vi "BorowskiMonitor.vi"() -> ()   [LabVIEW 2019]
uses:
  Utility/Monitor Communication/Brosowski/TempErrors.ctl
  Utility/Monitor Communication/Brosowski/TempErrors_in.ctl
  Utility/Monitor Communication/Brosowski/BorowskiMonitor.ctl
  Equipment/Mercury iXX/Public/Controls/Serial Settings.ctl
  Instrument_Setup.vi
  Equipment/Mercury iXX/Public/Libraries/System/Open/Open System.vi
  Global/Global Variables/Data_Display_global.vi
  Equipment/Mercury iXX/Mercury iXX.lvlib
  Equipment/Mercury iXX/Public/Libraries/Temperature.lvlib
  Equipment/Mercury iXX/Public/Libraries/Control Loop.lvlib
  Equipment/Mercury iXX/Public/Libraries/System.lvlib
panel:
  out "Borowski ITC-Cluster":T1 {"He3-Pot Heater %" format="%#_4g"; "He3-Pot Setpoint" format="%#_4g"; "Sorb Heater %" format="%#_4g"; "Sorb Setpoint" format="%#_4g"; "He3 Temp2" format="%#_4g"; "He3 Temp 1" format="%#_4g"; "1K Temp" format="%#_4g"; "Sorb Temp" format="%#_4g"}
  in  "Stop Monitoring":bool
  in  "TempErrorsIn":T2
  out "TempErrorsOut":T3
  in  "error in (no error)":errorcluster
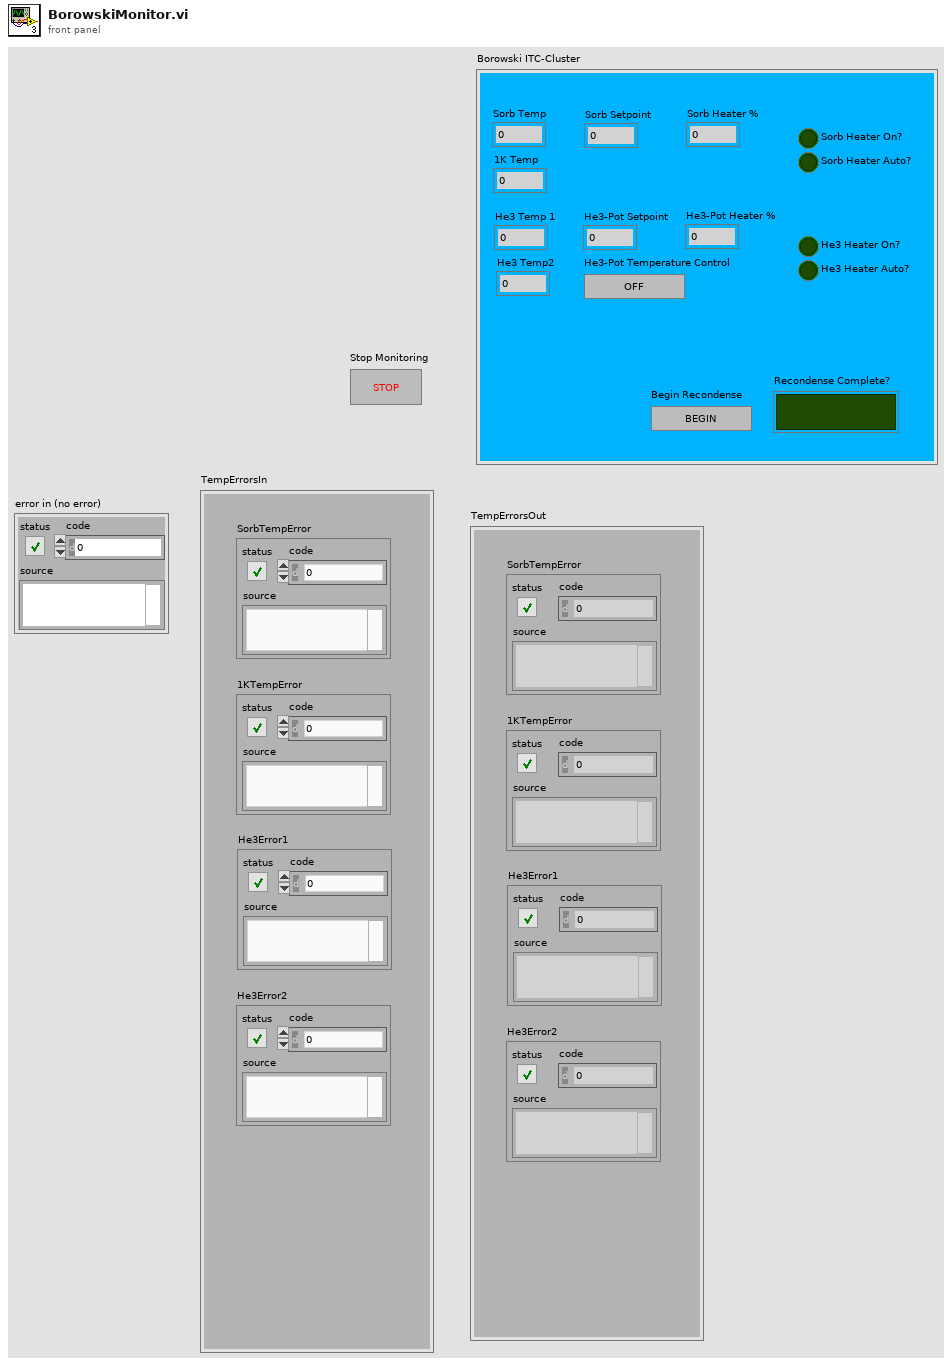
[diagram p1: front panel]
types:
  T1 = typedef "BorowskiMonitor.ctl" = cluster{"Sorb Temp":dbl, "1K Temp":dbl, "He3 Temp 1":dbl, "He3 Temp2":dbl, "Recondense Complete?":bool, "Sorb Heater Auto?":bool, "Sorb Heater On?":bool, "Sorb Setpoint":dbl, "Sorb Heater %":dbl, "Begin Recondense":bool, "He3-Pot Setpoint":dbl, "He3-Pot Heater %":dbl, "He3 Heater Auto?":bool, "He3 Heater On?":bool, "He3-Pot Temperature Control":bool}
  T2 = typedef "TempErrors_in.ctl" = cluster{"SorbTempError":errorcluster, "1KTempError":errorcluster, "He3Error1":errorcluster, "He3Error2":errorcluster}
  T3 = typedef "TempErrors.ctl" = cluster{"SorbTempError":errorcluster, "1KTempError":errorcluster, "He3Error1":errorcluster, "He3Error2":errorcluster}
  T4 = typedef "Mercury iXX.lvlib/Serial Settings.ctl" = cluster{"Baud Rate":u32, "Parity":u16, "Data Bits":u16, "Stop Bits":u16, "Flow Control":u16}
  T5 = typedef "Mercury iXX.lvlib/Comms Transport Layer.ctl" = enum16{"Ethernet TCP/IP", "USB", "ISOBus - RS-232", "GPIB"}
  T6 = cluster{"Comms Layer":T5, "IP Address":string, "VISA resource name":refnum<visa-resource-name>}
  T7 = typedef "Mercury iXX.lvlib/Mercury Reference.ctl" = cluster{"Comms":refnum<visa-resource-name>, "Device ID":string[], "Comms Layer":T5, "Command":string, "Query reference":T8}
  T8 = typedef "Mercury iXX.lvlib/Query Dynamic Reference.ctl" = refnum<vi>
  T9 = typedef "Borowski-Control-Cluster.ctl" = cluster{"Begin Recondense":bool, "Toggle He3-Pot Temperature Control":bool}
  T10 = typedef "Mercury_Reference_out.ctl" = cluster{"Mercury Reference In Sorb":T7, "Mercury Reference In 1K":T7, "Mercury Reference In H3 Temp1":T7, "Mercury Reference In H3 Temp2":T7}
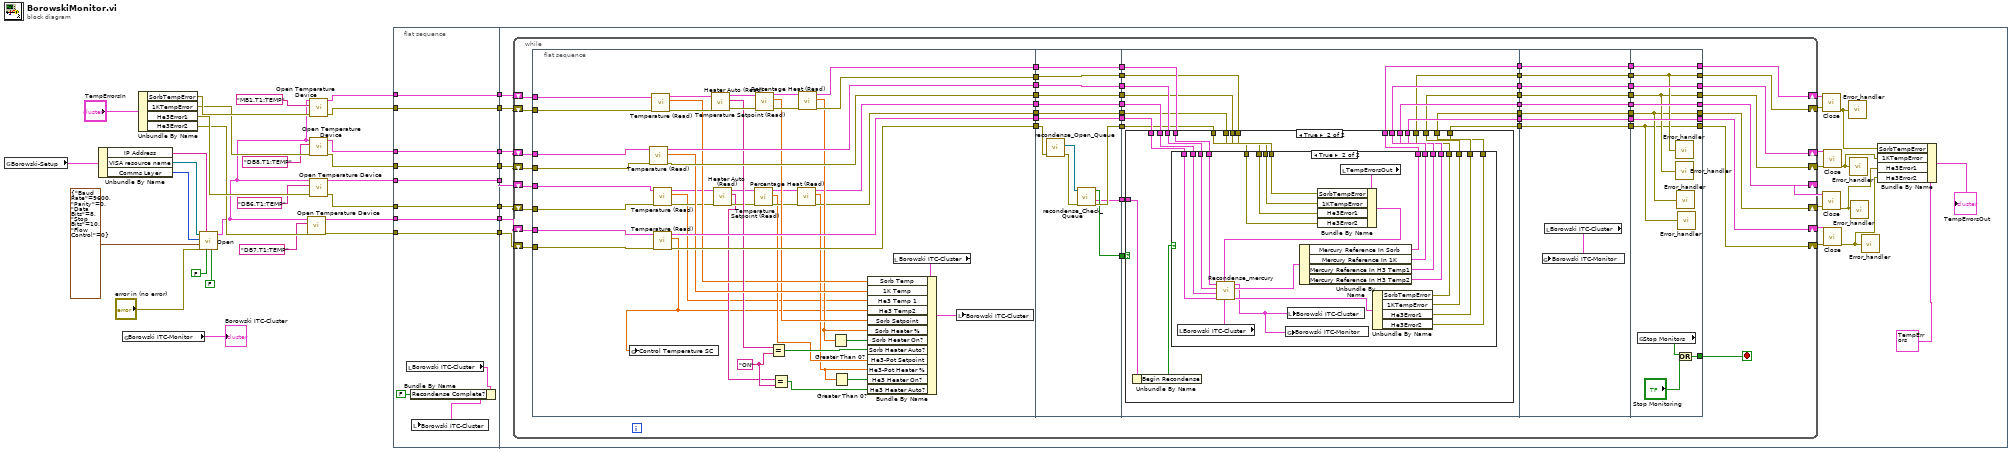
[diagram p0: block diagram]
diagram:
  n1 = global read "Instrument_Setup.vi" "Borowski-Setup"() -> (w14:T6)
  n2 = Unbundle By Name(w14) -> ("IP Address"=w13:string, "VISA resource name"=w12:refnum<visa-resource-name>, "Comms Layer"=w11:T5)
  n3 = global read "Data_Display_global.vi" "Borowski ITC-Monitor"() -> (→"Borowski ITC-Cluster":T1)
  n4 = Unbundle By Name("TempErrorsIn") -> ("SorbTempError"=w30:errorcluster, "1KTempError"=w29:errorcluster, "He3Error1"=w28:errorcluster, "He3Error2"=w27:errorcluster)
  n5 = call-poly "Open.vi"("Clear Previous Connections (False)"=FALSE, "ID Query (True)"=FALSE, "IP Address"=w13, "error in (no error)"="error in (no error)", "Serial Configuration"=T4 {"Baud Rate"=9600, "Parity"=0, "Data Bits"=8, "Stop Bits"=10, "Flow Control"=0}, "Comms Layer"=w11, "VISA resource name"=w12) -> ("Mercury Reference Out"=w1:T7)  [unwired: 4 out]
  n6 = call "Open Temperature Device.vi"("error in (no error)"=w27, "Device Identifier"="DB7.T1:TEMP", "Mercury Reference In"=w1) -> ("error out"=w18:errorcluster, "Mercury Reference Out"=w19:T7)  [unwired: 7 in]
  n7 = call "Open Temperature Device.vi"("error in (no error)"=w30, "Device Identifier"="MB1.T1:TEMP", "Mercury Reference In"=w1) -> ("error out"=w15:errorcluster, "Mercury Reference Out"=w22:T7)  [unwired: 7 in]
  n8 = call "Open Temperature Device.vi"("error in (no error)"=w29, "Device Identifier"="DB8.T1:TEMP", "Mercury Reference In"=w1) -> ("error out"=w16:errorcluster, "Mercury Reference Out"=w21:T7)  [unwired: 7 in]
  n9 = call "Open Temperature Device.vi"("error in (no error)"=w28, "Device Identifier"="DB6.T1:TEMP", "Mercury Reference In"=w1) -> ("error out"=w17:errorcluster, "Mercury Reference Out"=w20:T7)  [unwired: 7 in]
  n10 = flat-sequence {
    tunnel: w22 -> [w39]
    tunnel: w21 -> [w40]
    tunnel: w20 -> [w41]
    tunnel: w19 -> [w42]
    tunnel: w18 -> [w43]
    tunnel: w17 -> [w44]
    tunnel: w16 -> [w45]
    tunnel: w15 -> [w46]
    tunnel: [w46] -> w9
    tunnel: [w45] -> w8
    tunnel: [w44] -> w7
    tunnel: [w43] -> w6
    tunnel: [w42] -> w5
    tunnel: [w41] -> w4
    tunnel: [w40] -> w3
    tunnel: [w39] -> w2
    tunnel: w9 -> [w67]
    tunnel: w8 -> [w65]
    tunnel: w7 -> [w63]
    tunnel: w6 -> [w61]
    tunnel: w5 -> [w62]
    tunnel: w4 -> [w64]
    tunnel: w3 -> [w66]
    tunnel: w2 -> [w68]
    frame #0 {
      n11 = local read "Borowski ITC-Cluster"() -> (w38:T1)
      n12 = Bundle By Name(cluster=w38, "Recondense Complete?"=FALSE) -> (w37:T1)
      n13 = local write "Borowski ITC-Cluster"(w37) -> ()
    }
    frame #1 {
      n14 = while {
        shift-right: [w105] -> w60
        shift-left: w68 -> [w119]
        shift-right: [w117] -> w58
        shift-left: w66 -> [w118]
        shift-right: [w115] -> w56
        shift-left: w64 -> [w116]
        shift-right: [w113] -> w54
        shift-left: w62 -> [w114]
        shift-right: [w104] -> w59
        shift-left: w67 -> [w106]
        shift-right: [w107] -> w57
        shift-left: w65 -> [w108]
        shift-right: [w109] -> w55
        shift-left: w63 -> [w110]
        shift-right: [w111] -> w53
        shift-left: w61 -> [w112]
        stop <- w71 stop-if-true
        n15 = flat-sequence {
          tunnel: w119 -> [w164]
          tunnel: w118 -> [w163]
          tunnel: w116 -> [w161]
          tunnel: w114 -> [w160]
          tunnel: w112 -> [w158]
          tunnel: w110 -> [w156]
          tunnel: w108 -> [w155]
          tunnel: w106 -> [w153]
          tunnel: [w162] -> w103
          tunnel: [w122] -> w102
          tunnel: [w159] -> w101
          tunnel: [w157] -> w100
          tunnel: [w131] -> w99
          tunnel: [w154] -> w98
          tunnel: [w144] -> w97
          tunnel: [w143] -> w96
          tunnel: w103 -> [w177]
          tunnel: w102 -> [w176]
          tunnel: w101 -> [w175]
          tunnel: w100 -> [w170]
          tunnel: w99 -> [w174]
          tunnel: w98 -> [w173]
          tunnel: w97 -> [w172]
          tunnel: w96 -> [w171]
          tunnel: [w177] -> w95
          tunnel: [w176] -> w94
          tunnel: [w175] -> w93
          tunnel: [w168] -> w92
          tunnel: [w174] -> w91
          tunnel: [w173] -> w90
          tunnel: [w172] -> w89
          tunnel: [w171] -> w88
          tunnel: [w166] -> w70
          tunnel: [w165] -> w69
          tunnel: w95 -> [w192]
          tunnel: w94 -> [w190]
          tunnel: w93 -> [w188]
          tunnel: w92 -> [w180]
          tunnel: w91 -> [w182]
          tunnel: w90 -> [w184]
          tunnel: w89 -> [w194]
          tunnel: w88 -> [w186]
          tunnel: [w193] -> w87
          tunnel: [w191] -> w85
          tunnel: [w189] -> w83
          tunnel: [w181] -> w81
          tunnel: [w183] -> w79
          tunnel: [w185] -> w77
          tunnel: [w195] -> w75
          tunnel: [w187] -> w73
          tunnel: w70 -> [w179]
          tunnel: w69 -> [w178]
          tunnel: w87 -> [w260]
          tunnel: [w260] -> w86
          tunnel: w85 -> [w259]
          tunnel: [w259] -> w84
          tunnel: w83 -> [w258]
          tunnel: [w258] -> w82
          tunnel: w81 -> [w257]
          tunnel: [w257] -> w80
          tunnel: w79 -> [w256]
          tunnel: [w256] -> w78
          tunnel: w77 -> [w255]
          tunnel: [w255] -> w76
          tunnel: w75 -> [w254]
          tunnel: [w254] -> w74
          tunnel: w73 -> [w253]
          tunnel: [w253] -> w72
          tunnel: [w267] -> w104
          tunnel: [w268] -> w105
          tunnel: [w266] -> w107
          tunnel: [w265] -> w109
          tunnel: [w264] -> w111
          tunnel: [w269] -> w113
          tunnel: [w270] -> w115
          tunnel: [w271] -> w117
          tunnel: w86 -> [w271]
          tunnel: w84 -> [w270]
          tunnel: w82 -> [w269]
          tunnel: w80 -> [w264]
          tunnel: w78 -> [w265]
          tunnel: w76 -> [w266]
          tunnel: w74 -> [w268]
          tunnel: w72 -> [w267]
          tunnel: [w261] -> w71
          frame #0 {
            w128 = "ON" ("y")
            n16 = call "Temperature (Read).vi"("error in"=w155, "Mercury Reference In"=w163) -> ("error out"=w154:errorcluster, "Temperature"=w151:dbl, "Mercury Reference Out"=w162:T7)  [unwired: 5 in, 2 out]
            n17 = call "Temperature (Read).vi"("error in"=w153, "Mercury Reference In"=w164) -> ("error out"=w141:errorcluster, "Temperature"=w140:dbl, "Mercury Reference Out"=w142:T7)  [unwired: 5 in, 2 out]
            n18 = call "Temperature (Read).vi"("error in"=w156, "Mercury Reference In"=w161) -> ("error out"=w134:errorcluster, "Temperature"=w121:dbl, "Mercury Reference Out"=w135:T7)  [unwired: 5 in, 2 out]
            n19 = call "Temperature (Read).vi"("error in"=w158, "Mercury Reference In"=w160) -> ("error out"=w157:errorcluster, "Temperature"=w120:dbl, "Mercury Reference Out"=w159:T7)  [unwired: 5 in, 2 out]
            n20 = global write "Data_Display_global.vi" "Control Temperature SC"(w120) -> ()
            n21 = call "Heater Auto (Read).vi"("error in"=w141, "Mercury Reference In"=w142) -> ("error out"=w148:errorcluster, "Heater Auto"=w147:string, "Mercury Reference Out"=w149:T7)  [unwired: 6 in, 1 out]
            n22 = call "Heater Auto (Read).vi"("error in"=w134, "Mercury Reference In"=w135) -> ("error out"=w133:errorcluster, "Heater Auto"=w127:string, "Mercury Reference Out"=w130:T7)  [unwired: 6 in, 1 out]
            n23 = call "Temperature Setpoint (Read).vi"("error in"=w133, "Mercury Reference In"=w130) -> ("error out"=w132:errorcluster, "Temperature Setpoint"=w125:dbl, "Mercury Reference Out"=w129:T7)  [unwired: 5 in, 2 out]
            n24 = call "Temperature Setpoint (Read).vi"("error in"=w148, "Mercury Reference In"=w149) -> ("error out"=w145:errorcluster, "Temperature Setpoint"=w139:dbl, "Mercury Reference Out"=w146:T7)  [unwired: 5 in, 2 out]
            n25 = Equal?(x=w147, y=w128) -> (x = y?=w136:bool)
            n26 = Equal?(x=w127, y=w128) -> (x = y?=w126:bool)
            n27 = call "Percentage Heat (Read).vi"("error in"=w132, "Mercury Reference In"=w129) -> ("error out"=w131:errorcluster, "Percentage Heat"=w124:dbl, "Mercury Reference Out"=w122:T7)  [unwired: 5 in, 2 out]
            n28 = call "Percentage Heat (Read).vi"("error in"=w145, "Mercury Reference In"=w146) -> ("error out"=w143:errorcluster, "Percentage Heat"=w138:dbl, "Mercury Reference Out"=w144:T7)  [unwired: 5 in, 2 out]
            n29 = Greater Than 0?(x=w138) -> (x > 0?=w137:bool)
            n30 = Greater Than 0?(x=w124) -> (x > 0?=w123:bool)
            n31 = local read "Borowski ITC-Cluster"() -> (w152:T1)
            n32 = Bundle By Name(cluster=w152, "Sorb Temp"=w140, "1K Temp"=w151, "He3 Temp 1"=w121, "He3 Temp2"=w120, "Sorb Setpoint"=w139, "Sorb Heater %"=w138, "Sorb Heater On?"=w137, "Sorb Heater Auto?"=w136, "He3-Pot Setpoint"=w125, "He3-Pot Heater %"=w124, "He3 Heater On?"=w123, "He3 Heater Auto?"=w126) -> (w150:T1)
            n33 = local write "Borowski ITC-Cluster"(w150) -> ()
          }
          frame #1 {
            n34 = call "recondense_Open_Queue.vi"("error in (no error)"=w170) -> ("error out"=w169:errorcluster, "queue out"=w167:refnum<queue>)  [unwired: 9 in]
            n35 = call "recondense_Check_Queue.vi"("error in (no error)"=w169, "Queue"=w167) -> ("error out"=w168:errorcluster, "Recondense-Control"=w165:T9, "New Entries?"=w166:bool)  [unwired: 6 in]
          }
          frame #2 {
            n36 = case shown="True" w179 {
              tunnel: w194 -> [w199 w221]
              tunnel: [w199 w220] -> w195
              tunnel: w192 -> [w198 w219]
              tunnel: [w198 w218] -> w193
              tunnel: w190 -> [w197 w217]
              tunnel: [w197 w216] -> w191
              tunnel: w188 -> [w196 w215]
              tunnel: [w196 w214] -> w189
              tunnel: w186 -> [w203 w213]
              tunnel: w184 -> [w202 w212]
              tunnel: w182 -> [w201 w211]
              tunnel: w180 -> [w200 w210]
              tunnel: [w203 w209] -> w187
              tunnel: [w202 w208] -> w185
              tunnel: [w201 w207] -> w183
              tunnel: [w200 w206] -> w181
              tunnel: w178 -> [_ w205]
              frame False {
              }
              frame True {
                n37 = Unbundle By Name(w205) -> ("Begin Recondense"=w204:bool)
                n38 = case shown="True" w204 {
                  tunnel: w221 -> [w225 w249]
                  tunnel: [w225 w248] -> w220
                  tunnel: w219 -> [w224 w247]
                  tunnel: [w224 w246] -> w218
                  tunnel: w217 -> [w223 w245]
                  tunnel: [w223 w244] -> w216
                  tunnel: w215 -> [w222 w243]
                  tunnel: [w222 w242] -> w214
                  tunnel: w213 -> [w229 w239]
                  tunnel: w212 -> [w228 w238]
                  tunnel: w211 -> [w227 w237]
                  tunnel: w210 -> [w226 w236]
                  tunnel: [w229 w235] -> w209
                  tunnel: [w228 w234] -> w208
                  tunnel: [w227 w233] -> w207
                  tunnel: [w226 w232] -> w206
                  frame False {
                  }
                  frame True {
                    n39 = local read "Borowski ITC-Cluster"() -> (w231:T1)
                    n40 = local read "TempErrorsOut"() -> (w241:T3)
                    n41 = Bundle By Name(cluster=w241, "SorbTempError"=w239, "1KTempError"=w238, "He3Error1"=w237, "He3Error2"=w236) -> (w240:T3)
                    n42 = call "Recondense_mercury.vi"("Recondense-Monitor in"=w231, "TempErrorsIn"=w240, "Mercury Reference In H3 Temp2"=w243, "Mercury Reference In H3 Temp1"=w245, "Mercury Reference In 1K"=w247, "Mercury Reference In Sorb"=w249) -> ("TempErrorsOut"=w251:T3, "Mercury Reference out"=w250:T10, "Recondense-Monitor out"=w230:T1)  [unwired: 2 in]
                    n43 = global write "Data_Display_global.vi" "Borowski ITC-Monitor"(w230) -> ()
                    n44 = local write "Borowski ITC-Cluster"(w230) -> ()
                    n45 = Unbundle By Name(w250) -> ("Mercury Reference In Sorb"=w248:T7, "Mercury Reference In 1K"=w246:T7, "Mercury Reference In H3 Temp1"=w244:T7, "Mercury Reference In H3 Temp2"=w242:T7)
                    n46 = Unbundle By Name(w251) -> ("SorbTempError"=w235:errorcluster, "1KTempError"=w234:errorcluster, "He3Error1"=w233:errorcluster, "He3Error2"=w232:errorcluster)
                  }
                }
              }
            }
          }
          frame #3 {
            n47 = local read "Borowski ITC-Cluster"() -> (w252:T1)
            n48 = global write "Data_Display_global.vi" "Borowski ITC-Monitor"(w252) -> ()
          }
          frame #4 {
            n49 = global read "Data_Display_global.vi" "Stop Monitors"() -> (w262:bool)
            n50 = call "Error_handler.vi"("error constant"=w267) -> ()
            n51 = call "Error_handler.vi"("error constant"=w266) -> ()
            n52 = call "Error_handler.vi"("error constant"=w265) -> ()
            n53 = Or(x=w262, y="Stop Monitoring") -> (x .or. y?=w261:bool)
            n54 = call "Error_handler.vi"("error constant"=w264) -> ()
          }
        }
      }
      n55 = call "Close.vi"("error in (no error)"=w59, "Mercury Reference"=w60) -> ("error out"=w50:errorcluster)  [unwired: 9 in]
      n56 = call "Close.vi"("error in (no error)"=w55, "Mercury Reference"=w56) -> ("error out"=w48:errorcluster)  [unwired: 9 in]
      n57 = call "Close.vi"("error in (no error)"=w57, "Mercury Reference"=w58) -> ("error out"=w49:errorcluster)  [unwired: 9 in]
      n58 = call "Close.vi"("error in (no error)"=w53, "Mercury Reference"=w54) -> ("error out"=w47:errorcluster)  [unwired: 9 in]
      n59 = call "Error_handler.vi"("error constant"=w50) -> ()
      n60 = call "Error_handler.vi"("error constant"=w49) -> ()
      n61 = call "Error_handler.vi"("error constant"=w48) -> ()
      n62 = call "Error_handler.vi"("error constant"=w47) -> ()
      n63 = Bundle By Name(cluster=T3 {"SorbTempError"={"status"=FALSE, "code"=0, "source"=""}, "1KTempError"={"status"=FALSE, "code"=0, "source"=""}, "He3Error1"={"status"=FALSE, "code"=0, "source"=""}, "He3Error2"={"status"=FALSE, "code"=0, "source"=""}} ("TempErrorsOut"), "SorbTempError"=w50, "1KTempError"=w49, "He3Error1"=w48, "He3Error2"=w47) -> (→"TempErrorsOut":T3)
    }
  }
